vi "Run_Core.vi"(0 "String Operations in":refnum<class "String Operations.lvclass">, 11 "error in (no error)":errorcluster) -> (4 "String Operations out":refnum<class "String Operations.lvclass">, 6 "Return":variant, 15 "error out":errorcluster)   [LabVIEW 2016, in "String Operations.lvclass"]
uses:
  String Operations.lvclass
  D:/TOOLS/LSL/source code/LSL components/functions/functionsbase/functionbase.lvclass
  functionsbase/functionbase.lvclass/functionbase.ctl
  String Operations.lvclass/String Operations.ctl
  functionsbase/properties/Read Smart Syntax Representation.vi
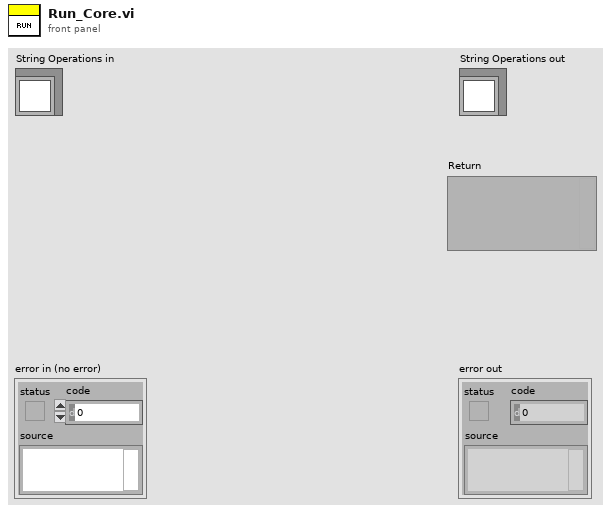
[diagram p1: front panel]
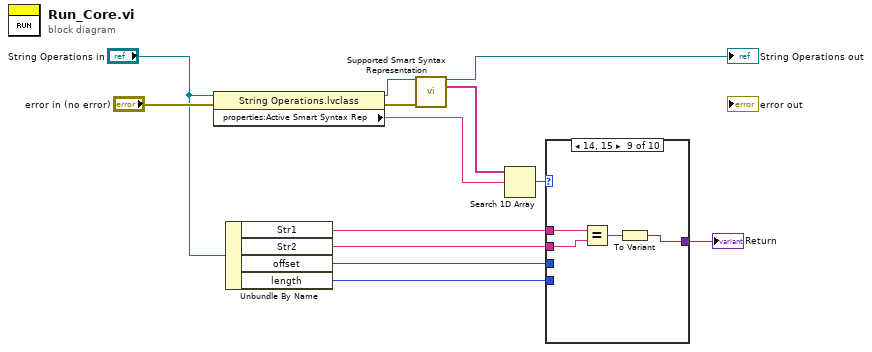
[diagram p0: block diagram]
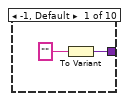
[diagram p2: hidden frame]
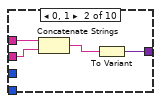
[diagram p3: hidden frame]
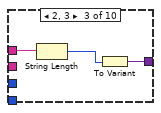
[diagram p4: hidden frame]
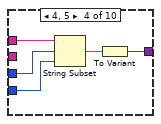
[diagram p5: hidden frame]
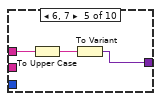
[diagram p6: hidden frame]
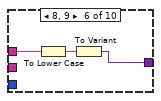
[diagram p7: hidden frame]
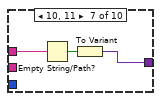
[diagram p8: hidden frame]
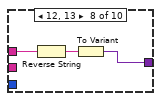
[diagram p9: hidden frame]
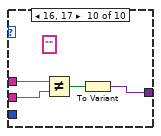
[diagram p10: hidden frame]
diagram:
  n1 = property class="String Operations.lvclass"(reference="String Operations in", error in="error in (no error)") -> (reference out=w9:refnum<class "String Operations.lvclass">, error out=w12:errorcluster, "properties:Active Smart Syntax Rep"=w6:string)
  n2 = Unbundle By Name("String Operations in") -> ("Str1"=w5:string, "Str2"=w4:string, "offset"=w2:i32, "length"=w1:i32)
  n3 = call-dynamic "Supported Smart Syntax Representation.vi"("String Operations in"=w9, "error in (no error)"=w12) -> ("String Operations out"=→"String Operations out":refnum<class "String Operations.lvclass">, "Smart Syntax Representation List"=w11:string[])  [unwired: 11 in, 1 out]
  n4 = Search 1D Array(1D array=w11, element=w6) -> (index of element=w10:i32)  [unwired: 1 in]
  n5 = case shown="14, 15" w10 {
    tunnel: w5 -> [_ w19 w22 w27 w30 w33 w36 w39 w43 w47]
    tunnel: w4 -> [_ w18 _ _ _ _ _ _ w42 w46]
    tunnel: [w14 w16 w20 w23 w28 w31 w35 w37 w41 w45] -> w3
    tunnel: w2 -> [_ _ _ w26 _ _ _ _ _ _]
    tunnel: w1 -> [_ _ _ w25 _ _ _ _ _ _]
    frame -1, Default {
      n6 = To Variant(anything="") -> (Variant=w14:variant)
    }
    frame 0, 1 {
      n7 = Concatenate Strings(w19, w18) -> (w17:string)
      n8 = To Variant(anything=w17) -> (Variant=w16:variant)
    }
    frame 2, 3 {
      n9 = String Length(string=w22) -> (length=w21:i32)
      n10 = To Variant(anything=w21) -> (Variant=w20:variant)
    }
    frame 4, 5 {
      n11 = String Subset(string=w27, offset (0)=w26, length (rest)=w25) -> (substring=w24:string)
      n12 = To Variant(anything=w24) -> (Variant=w23:variant)
    }
    frame 6, 7 {
      n13 = To Upper Case(1:w30) -> (0:w29:string)
      n14 = To Variant(anything=w29) -> (Variant=w28:variant)
    }
    frame 8, 9 {
      n15 = To Lower Case(string=w33) -> (all lower case string=w32:string)
      n16 = To Variant(anything=w32) -> (Variant=w31:variant)
    }
    frame 10, 11 {
      n17 = Empty String/Path?(string/path=w36) -> (empty?=w34:bool)
      n18 = To Variant(anything=w34) -> (Variant=w35:variant)
    }
    frame 12, 13 {
      n19 = Reverse String(1:w39) -> (0:w38:string)
      n20 = To Variant(anything=w38) -> (Variant=w37:variant)
    }
    frame 14, 15 {
      n21 = Equal?(x=w43, y=w42) -> (x = y?=w40:bool)
      n22 = To Variant(anything=w40) -> (Variant=w41:variant)
    }
    frame 16, 17 {
      (unwired) ""
      n23 = Not Equal?(x=w47, y=w46) -> (x != y?=w44:bool)
      n24 = To Variant(anything=w44) -> (Variant=w45:variant)
    }
  }
  "Return" <- w3
